vi "CALCULATOR VI PROGRAM.vi"() -> ()   [LabVIEW 2015]
panel:
  in  "stop":bool
  in  "Calculator UI":T1
  out "Calculator Display":string
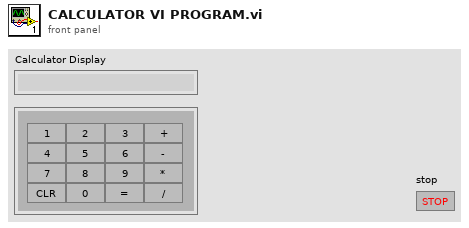
[diagram p1: front panel]
types:
  T1 = cluster{"1":bool, "2":bool, "3":bool, "Add":bool, "4":bool, "5":bool, "6":bool, "Subtract":bool, "7":bool, "8":bool, "9":bool, "Result":bool, "Clear":bool, "0":bool, "Multiply":bool, "Divide":bool}
  T2 = enum16{"Div", "Mul", "Sub", "Add", "No function"}
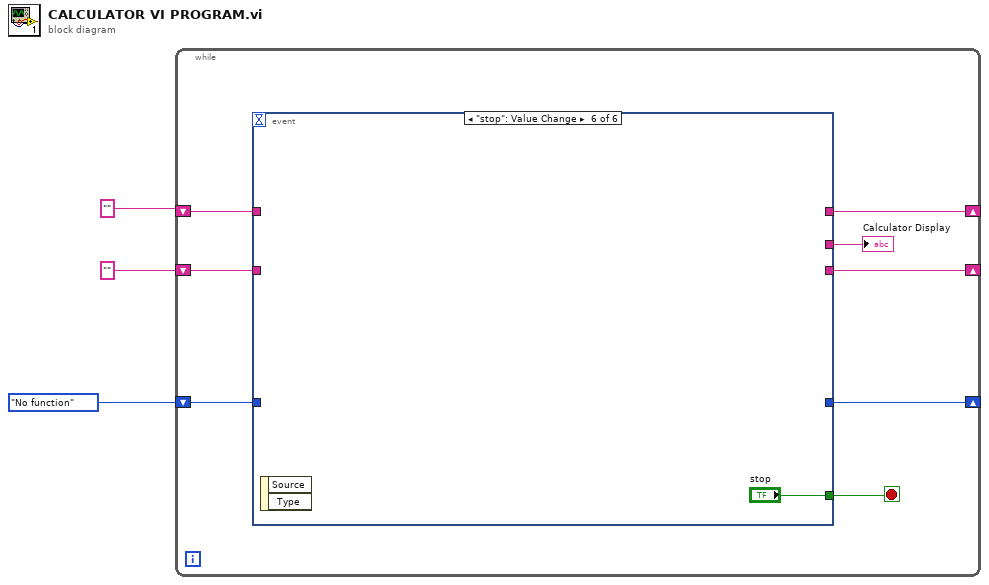
[diagram p0: block diagram]
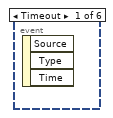
[diagram p2: hidden frame]
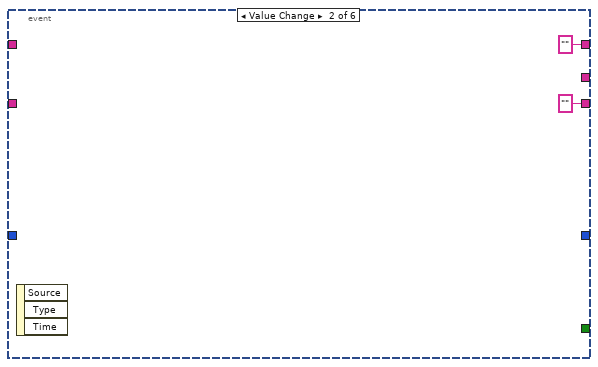
[diagram p3: hidden frame]
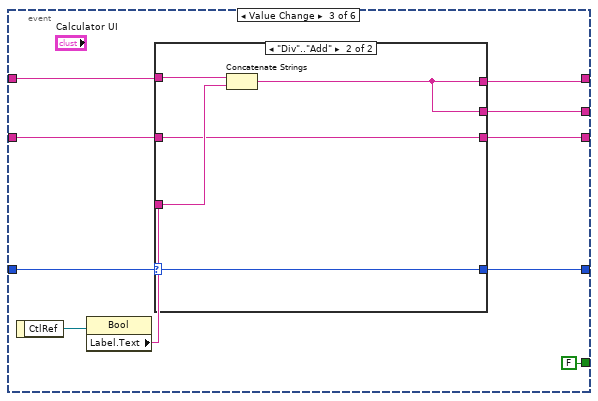
[diagram p4: hidden frame]
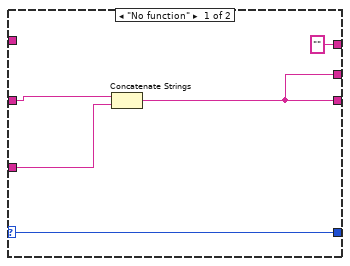
[diagram p5: hidden frame]
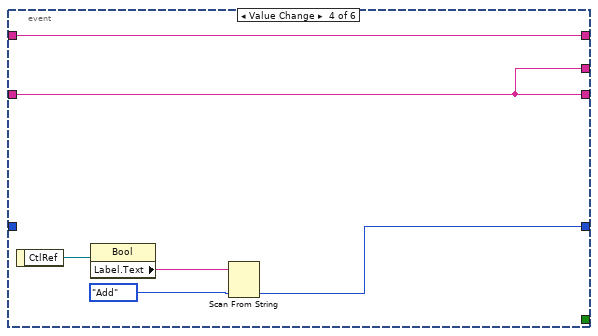
[diagram p6: hidden frame]
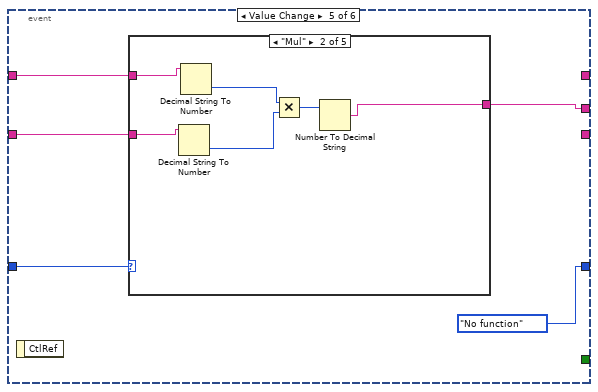
[diagram p7: hidden frame]
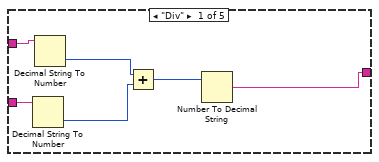
[diagram p8: hidden frame]
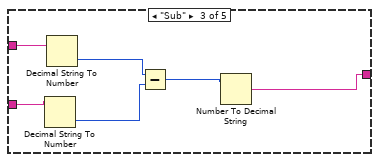
[diagram p9: hidden frame]
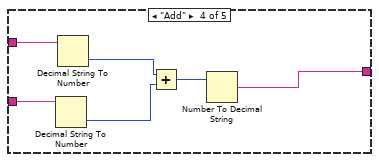
[diagram p10: hidden frame]
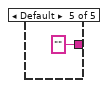
[diagram p11: hidden frame]
diagram:
  n1 = while {
    shift-right: [w9] -> _
    shift-left: T2."No function" -> [w10]
    shift-right: [w6] -> _
    shift-left: "" -> [w11]
    shift-right: [w7] -> _
    shift-left: "" -> [w8]
    stop <- w4 stop-if-true
    n2 = event shown="[5] \"stop\": Value Change" {
      selector: _ -> [_ _ _ _ _ _]
      dyn-events: _ -> [_ _ _ _ _ _]
      timeout: _ -> [_ _ _ _ _ _]
      tunnel: w11 -> [_ _ w21 w35 w43 _]
      tunnel: w10 -> [_ _ w22 _ w44 _]
      tunnel: [_ _ w14 w36 T2."No function" _] -> w9
      tunnel: [_ "" w16 w35 _ _] -> w6
      tunnel: [_ "" w17 w34 _ _] -> w7
      tunnel: w8 -> [_ _ w18 w34 w42 _]
      tunnel: [_ _ w15 w34 w41 _] -> w5
      tunnel: [_ _ FALSE _ _ "stop"] -> w4
      event Timeout {
        n3 = event-data() -> ()  [unwired: 1 in, 3 out]
      }
      event "Calculator UI.Clear": Value Change {
        n4 = event-data() -> ()  [unwired: 1 in, 3 out]
      }
      event "Calculator UI.0", "Calculator UI.2", "Calculator UI.3", "Calculator UI.4", "Calculator UI.5", "Calculator UI.6", "Calculator UI.7", "Calculator UI.8", "Calculator UI.9": Value Change {
        n5 = event-data() -> ("CtlRef"=w23:refnum<vi>)  [unwired: 1 in]
        n6 = property class="Bool"(reference=w23) -> ("Label.Text"=w20:string)  [unwired: 1 in, 2 out]
        n7 = case shown="\"Div\"..\"Add\"" w22 {
          selector: w22 -> [w24 w29]
          tunnel: w21 -> [_ w33]
          tunnel: w20 -> [w28 w32]
          tunnel: w18 -> [w27 w30]
          tunnel: [w25 w30] -> w17
          tunnel: ["" w31] -> w16
          tunnel: [w25 w31] -> w15
          tunnel: [w24 w29] -> w14
          frame "No function" {
            n8 = Concatenate Strings(w27, w28) -> (w25:string)
          }
          frame "Div".."Add" {
            n9 = Concatenate Strings(w33, w32) -> (w31:string)
          }
        }
      }
      event "Calculator UI.Add", "Calculator UI.Subtract", "Calculator UI.Multiply", "Calculator UI.Divide": Value Change {
        n10 = event-data() -> ("CtlRef"=w39:refnum<vi>)  [unwired: 1 in]
        n11 = property class="Bool"(reference=w39) -> ("Label.Text"=w38:string)  [unwired: 1 in, 2 out]
        n12 = Scan From String(input string=w38, default 1=T2."Add") -> (output 1=w36:T2)  [unwired: 3 in, 3 out]
      }
      event "Calculator UI.Result": Value Change {
        n13 = event-data() -> ()  [unwired: 1 in, 1 out]
        n14 = case shown="\"Mul\"" w44 {
          tunnel: w43 -> [w48 w54 w60 w68 _]
          tunnel: w42 -> [w47 w53 w59 w67 _]
          tunnel: [w46 w52 w58 w64 ""] -> w41
          frame "Div" {
            n15 = Decimal String To Number(string=w47) -> (number=w50:i32)  [unwired: 2 in, 1 out]
            n16 = Decimal String To Number(string=w48) -> (number=w49:i32)  [unwired: 2 in, 1 out]
            n17 = Add(x=w49, y=w50) -> (x+y=w45:i32)
            n18 = Number To Decimal String(number=w45) -> (decimal integer string=w46:string)  [unwired: 1 in]
          }
          frame "Mul" {
            n19 = Decimal String To Number(string=w53) -> (number=w56:i32)  [unwired: 2 in, 1 out]
            n20 = Decimal String To Number(string=w54) -> (number=w55:i32)  [unwired: 2 in, 1 out]
            n21 = Multiply(x=w55, y=w56) -> (x*y=w51:i32)
            n22 = Number To Decimal String(number=w51) -> (decimal integer string=w52:string)  [unwired: 1 in]
          }
          frame "Sub" {
            n23 = Decimal String To Number(string=w59) -> (number=w62:i32)  [unwired: 2 in, 1 out]
            n24 = Decimal String To Number(string=w60) -> (number=w61:i32)  [unwired: 2 in, 1 out]
            n25 = Subtract(x=w61, y=w62) -> (x-y=w57:i32)
            n26 = Number To Decimal String(number=w57) -> (decimal integer string=w58:string)  [unwired: 1 in]
          }
          frame "Add" {
            n27 = Decimal String To Number(string=w67) -> (number=w66:i32)  [unwired: 2 in, 1 out]
            n28 = Decimal String To Number(string=w68) -> (number=w65:i32)  [unwired: 2 in, 1 out]
            n29 = Add(x=w65, y=w66) -> (x+y=w63:i32)
            n30 = Number To Decimal String(number=w63) -> (decimal integer string=w64:string)  [unwired: 1 in]
          }
          frame Default {
          }
        }
      }
      event "stop": Value Change {
        n31 = event-data() -> ()  [unwired: 1 in, 2 out]
      }
    }
    "Calculator Display" <- w5
  }
